vi "Que_Temp.vi"(6 "TimeOut(5000)":i32=5000, 8 "error in":errorcluster, 10 "Event":string, 11 "TargetQName":string) -> (0 "error out":errorcluster, 1 "timed out":bool caption="Time Out?", 2 "Data":variant, 3 "Event out":string)   [LabVIEW 2016]
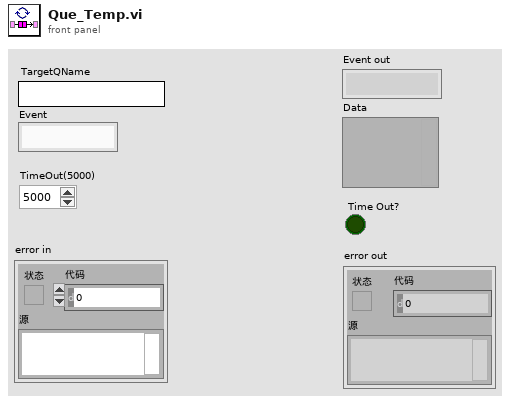
[diagram p1: front panel]
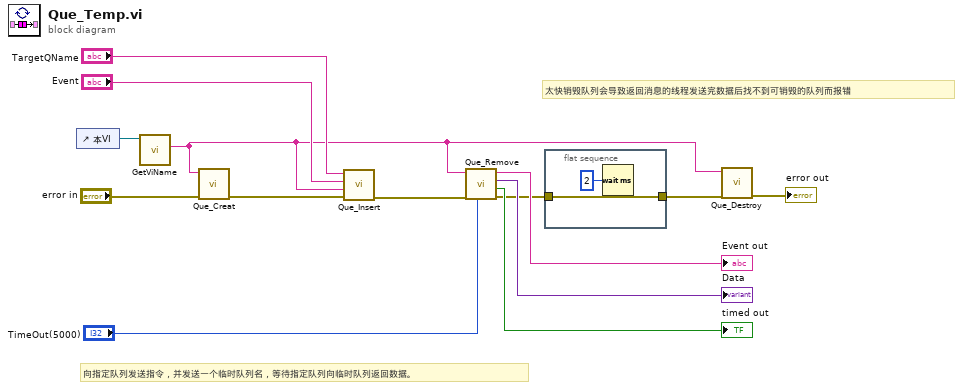
[diagram p0: block diagram]
diagram:
  # "太快销毁队列会导致返回消息的线程发送完数据后找不到可销毁的队列而报错"
  # "向指定队列发送指令，并发送一个临时队列名，等待指定队列向临时队列返回数据。"
  n1 = control-ref of="本VI"() -> (w14:refnum<vi>)
  n2 = call "GetViName.vi"("VI*"=w14) -> ("VI Name"=w8:string)  [unwired: 9 in, 1 out]
  n3 = call "Que_Creat.vi"("error in (no error)"="error in", "QueueName"=w8) -> ("error out"=w13:errorcluster)  [unwired: 8 in, 1 out]
  n4 = call "Que_Insert.vi"("error in"=w13, "Data"=w8, "Event"="Event", "QueueName"="TargetQName") -> ("error out"=w10:errorcluster)  [unwired: 6 in, 1 out]
  n5 = call "Que_Remove.vi"("Time out(-1)"="TimeOut(5000)", "error in (no error)"=w10, "Queue Name"=w8) -> ("error out"=w2:errorcluster, "timed out"=→"timed out":bool, "Data"=→"Data":variant, "Event"=→"Event out":string)  [unwired: 5 in]
  n6 = flat-sequence {
    tunnel: w2 -> [w16]
    tunnel: [w16] -> w1
    frame #0 {
      n7 = Wait (ms)(milliseconds to wait=u32 2 ("等待时间（毫秒）")) -> ()  [unwired: 1 out]
    }
  }
  n8 = call "Que_Destroy.vi"("error in (no error)"=w1, "QueeuName"=w8) -> ("error out"=→"error out":errorcluster)  [unwired: 9 in]
